vi "Read results object lookup string array.vi"(8 "error in (no error)":errorcluster, 11 "UI in":refnum<class "UI.lvclass">) -> (0 "error out":errorcluster, 2 "results object lookup string array":string[](array[string]), 3 "UI out":refnum<class "UI.lvclass">)   [LabVIEW 2016, in "Generic UI Actor.lvlib" / "UI.lvclass"]
uses:
  <userlib>/Common Components/User Interface/UI.lvclass
  <userlib>/Common Components/User Interface/UI.lvclass/UI.ctl
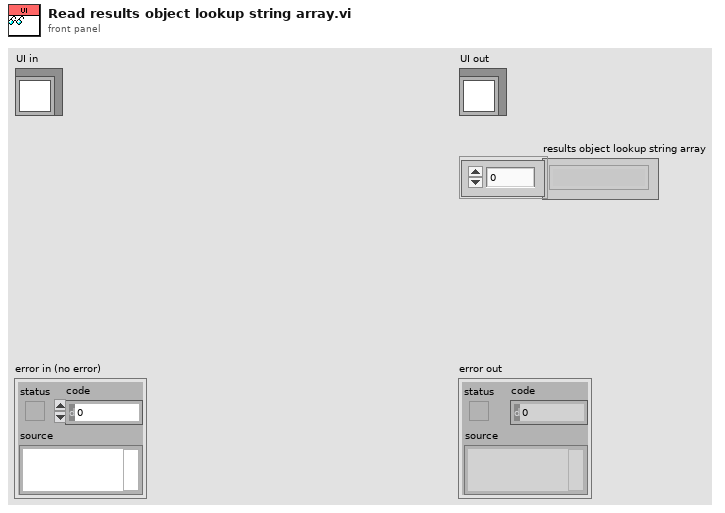
[diagram p1: front panel]
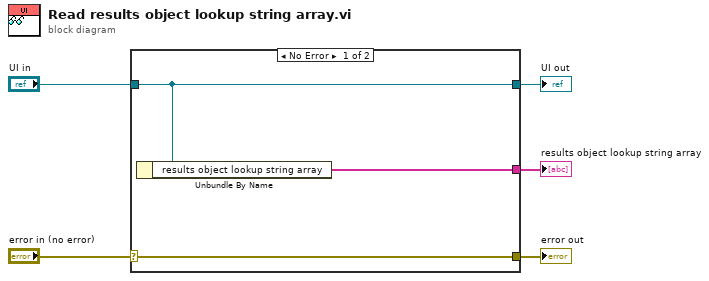
[diagram p0: block diagram]
diagram:
  n1 = case shown="No Error" "error in (no error)" {
    selector: "error in (no error)" -> [w8 w9]
    tunnel: [w8 w9] -> w4
    tunnel: [w7 w10] -> w2
    tunnel: "UI in" -> [w7 w10]
    tunnel: [w6 _] -> w1
    frame No Error {
      n2 = Unbundle By Name(w7) -> ("results object lookup string array"=w6:string[])
    }
    frame Error {
    }
  }
  "error out" <- w4
  "UI out" <- w2
  "results object lookup string array" <- w1
